vi "Calculate Point Cloud Distance.vi"(8 "error in (no error)":errorcluster, 10 "Moving point cloud":cluster{"X":sgl, "Y":sgl}[](array[cluster]), 11 "Fixed point cloud":cluster{"X":sgl, "Y":sgl}[](array[cluster])) -> (0 "error out":errorcluster, 1 "Alignment quality":sgl, 2 "y displacement":sgl, 3 "x displacement":sgl)   [LabVIEW 2012]
uses:
  <vilib>/Analysis/baseanly.llb/Mean (DBL).vi
  <vilib>/Analysis/NI_AALBase.lvlib
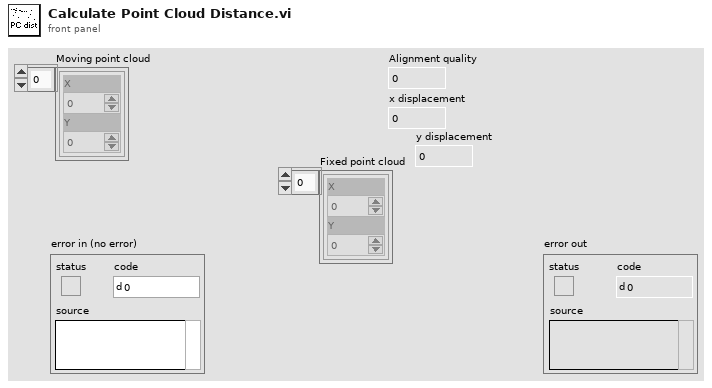
[diagram p1: front panel]
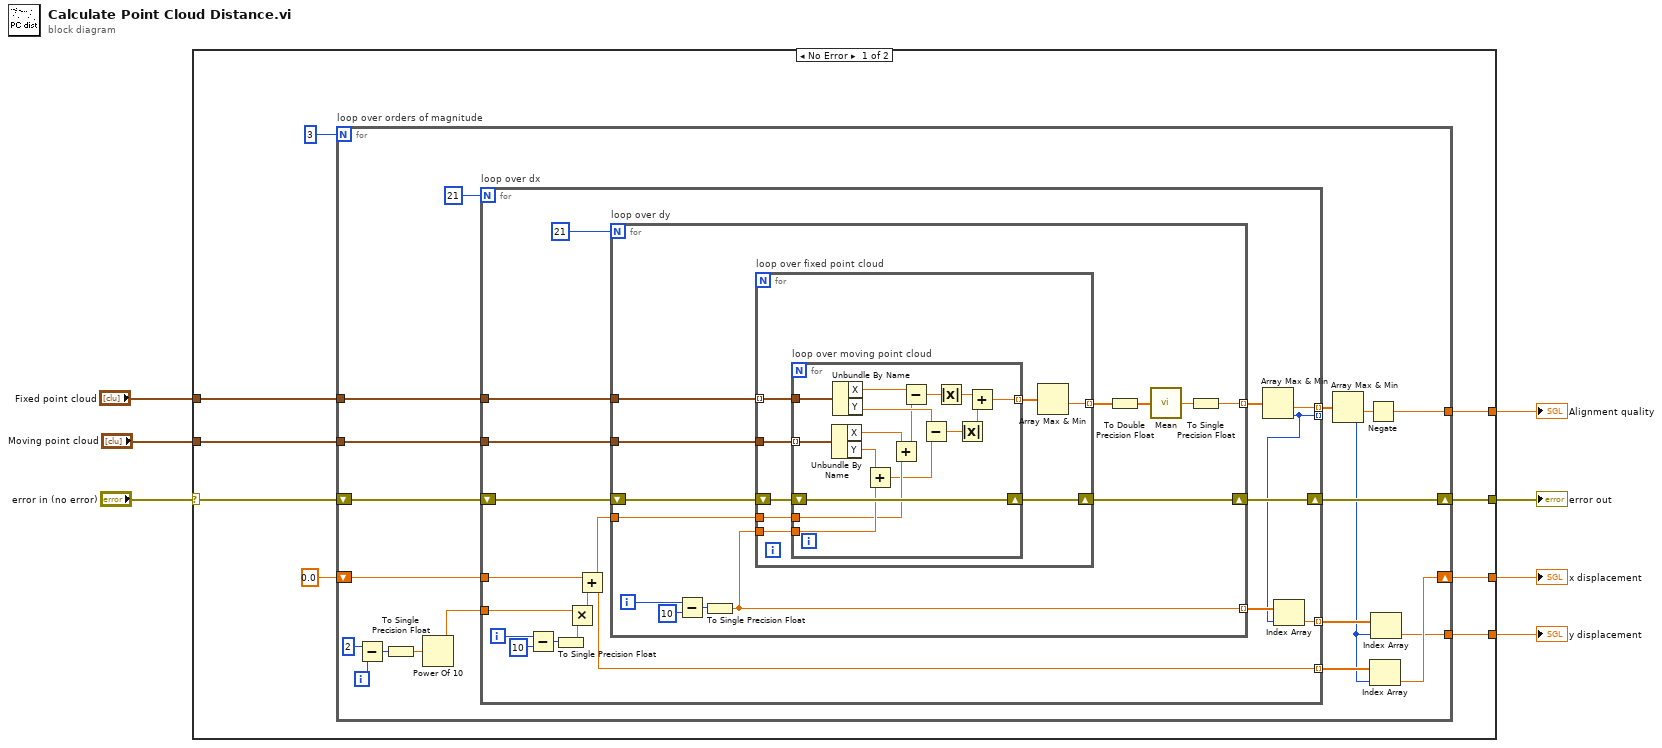
[diagram p0: block diagram]
diagram:
  n1 = case shown="No Error" "error in (no error)" {
    selector: "error in (no error)" -> [w13 w91]
    tunnel: [w12 w91] -> w6
    tunnel: "Fixed point cloud" -> [w15 _]
    tunnel: "Moving point cloud" -> [w14 _]
    tunnel: [w10 _] -> w3
    tunnel: [w9 _] -> w1
    tunnel: [w8 _] -> w2
    frame No Error {
      n2 = for "loop over orders of magnitude" {
        N: 3 -> [_]
        tunnel: w15 -> [w33]
        tunnel: w14 -> [w32]
        shift-right: [w30] -> w12
        shift-left: w13 -> [w31]
        tunnel: [w17] -> w8
        shift-right: [w27] -> w10
        shift-left: sgl 0.0 ("x") -> [w26]
        tunnel: [w23] -> w9
        i -> [w20]
        n3 = Subtract(x=2, y=w20) -> (x-y=w18:i32)
        n4 = To Single Precision Float(number=w18) -> (single precision float=w35:sgl)
        n5 = Power Of 10(x=w35) -> (10^x=w21:sgl)
        n6 = for "loop over dx" {
          N: 21 -> [_]
          tunnel: w21 -> [w48]
          tunnel: w33 -> [w47]
          tunnel: w32 -> [w46]
          shift-right: [w44] -> w30
          shift-left: w31 -> [w45]
          tunnel: [w40] -> w29 mode=indexing
          tunnel: [w38] -> _ mode=indexing
          tunnel: [w37] -> w25 mode=indexing
          tunnel: [w36] -> w28 mode=indexing
          tunnel: w26 -> [w42]
          i -> [w52]
          n7 = Subtract(x=w52, y=10) -> (x-y=w50:i32)
          n8 = To Single Precision Float(number=w50) -> (single precision float=w49:sgl)
          n9 = Multiply(x=w48, y=w49) -> (x*y=w43:sgl)
          n10 = Add(x=w42, y=w43) -> (x+y=w36:sgl)
          n11 = for "loop over dy" {
            N: 21 -> [_]
            tunnel: w47 -> [w63]
            tunnel: w46 -> [w62]
            shift-right: [w60] -> w44
            shift-left: w45 -> [w61]
            tunnel: w36 -> [w59]
            tunnel: [w54] -> w41 mode=indexing
            tunnel: [w57] -> w39 mode=indexing
            i -> [w64]
            n12 = Subtract(x=w64, y=10) -> (x-y=w66:i32)
            n13 = To Single Precision Float(number=w66) -> (single precision float=w57:sgl)
            n14 = for "loop over fixed point cloud" {
              tunnel: w63 -> [w74] mode=indexing
              tunnel: w62 -> [w73]
              shift-right: [w71] -> w60
              shift-left: w61 -> [w72]
              tunnel: w57 -> [w70]
              tunnel: w59 -> [w69]
              tunnel: [w67] -> w56 mode=indexing
              n15 = for "loop over moving point cloud" {
                tunnel: w74 -> [w89]
                tunnel: w73 -> [w88] mode=indexing
                shift-right: [w90] -> w71
                shift-left: w72 -> [w90]
                tunnel: w70 -> [w86]
                tunnel: w69 -> [w84]
                tunnel: [w75] -> w68 mode=indexing
                n16 = Unbundle By Name(w88) -> ("X"=w85:sgl, "Y"=w87:sgl)
                n17 = Unbundle By Name(w89) -> ("X"=w80:sgl, "Y"=w82:sgl)
                n18 = Add(x=w87, y=w86) -> (x+y=w83:sgl)
                n19 = Add(x=w85, y=w84) -> (x+y=w81:sgl)
                n20 = Subtract(x=w80, y=w81) -> (x-y=w79:sgl)
                n21 = Subtract(x=w82, y=w83) -> (x-y=w78:sgl)
                n22 = Absolute Value(x=w79) -> (abs(x)=w76:sgl)
                n23 = Absolute Value(x=w78) -> (abs(x)=w77:sgl)
                n24 = Add(x=w76, y=w77) -> (x+y=w75:sgl)
              }
              n25 = Array Max & Min(array=w68) -> (min value=w67:sgl)  [unwired: 3 out]
            }
            n26 = To Double Precision Float(number=w56) -> (double precision float=w55:dbl[])
            n27 = call-poly <vilib>:"Mean.vi"("X"=w55) -> ("mean"=w58:dbl)  [unwired: 1 out]
            n28 = To Single Precision Float(number=w58) -> (single precision float=w54:sgl)
          }
          n29 = Array Max & Min(array=w41) -> (min value=w40:sgl, min index (indices)=w38:i32)  [unwired: 2 out]
          n30 = Index Array(array=w39, index=w38) -> (element=w37:sgl)
        }
        n31 = Array Max & Min(array=w29) -> (min value=w22:sgl, min index (indices)=w24:i32)  [unwired: 2 out]
        n32 = Negate(x=w22) -> (-x=w17:sgl)
        n33 = Index Array(array=w28, index=w24) -> (element=w27:sgl)
        n34 = Index Array(array=w25, index=w24) -> (element=w23:sgl)
      }
    }
    frame Error {
    }
  }
  "error out" <- w6
  "Alignment quality" <- w2
  "x displacement" <- w3
  "y displacement" <- w1
